vi "calculate_scanner_delays.vi"(8 "error in (no error)":errorcluster, 9 "position feedback data":T2, 10 "transformation parameters":T1={"scale factor"=1.0, "rotation angle"=0.0, "tilting angle"=0.0, "offset"=refnum}, 11 "TrajectoryDL091126GenericVoxel in":refnum<class "TrajectoryDL091126GenericVoxel.lvclass">) -> (0 "error out":errorcluster, 2 "calculated scanner delays":i32[](array[numeric]), 3 "TrajectoryDL091126GenericVoxel out":refnum<class "TrajectoryDL091126GenericVoxel.lvclass">)   [LabVIEW 2010, in "TrajectoryDL091126GenericVoxel.lvclass"]
uses:
  TrajectoryDL091126GenericVoxel.lvclass
  common/arrays/pixel_raw_data_array.ctl
  transformation_parameters.ctl
  common/classes/SpaceVector/SpaceVector/SpaceVector.lvclass
  <vilib>/Analysis/2dsp.llb/1D Cross Correlation (DBL).vi
  common/classes/ErrorController/ErrorController/class_data.vi
  <vilib>/Analysis/NI_AALPro.lvlib
  common/classes/ErrorController/ErrorController/ErrorController.lvclass
panel:
  out "Z scanner":dbl[](graph)
  out "Y scanner":dbl[](graph)
  out "X scanner":dbl[](graph)
  # "This VI uses cross-correlation to calculate the scanner delay.\n\nOverwrite this method in your Trajectory child class if you want to have your own algorithm."
  # "Cross-correlations between command and position-feedback signals"
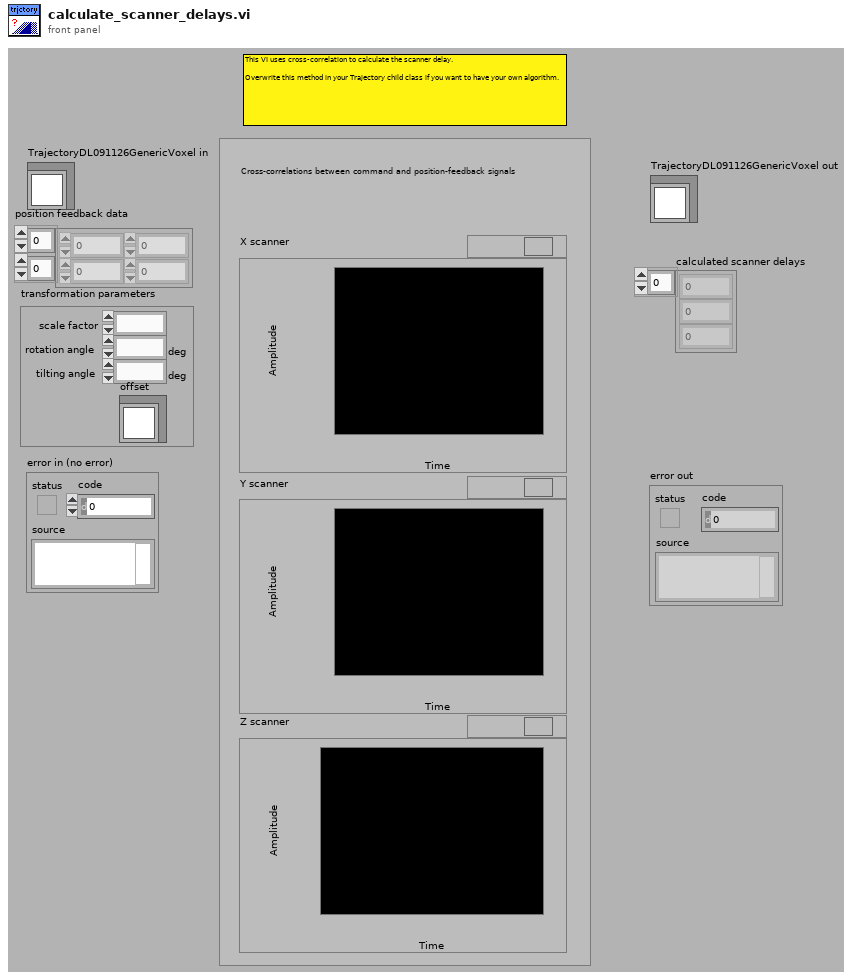
[diagram p1: front panel]
types:
  T1 = typedef "TrajectoryDL091126GenericVoxel.lvclass/transformation_parameters.ctl" = cluster{"scale factor":dbl, "rotation angle":dbl[unit], "tilting angle":dbl[unit], "offset":refnum<class "SpaceVector.lvclass">}
  T2 = typedef "pixel_raw_data_array.ctl" = dbl[][]
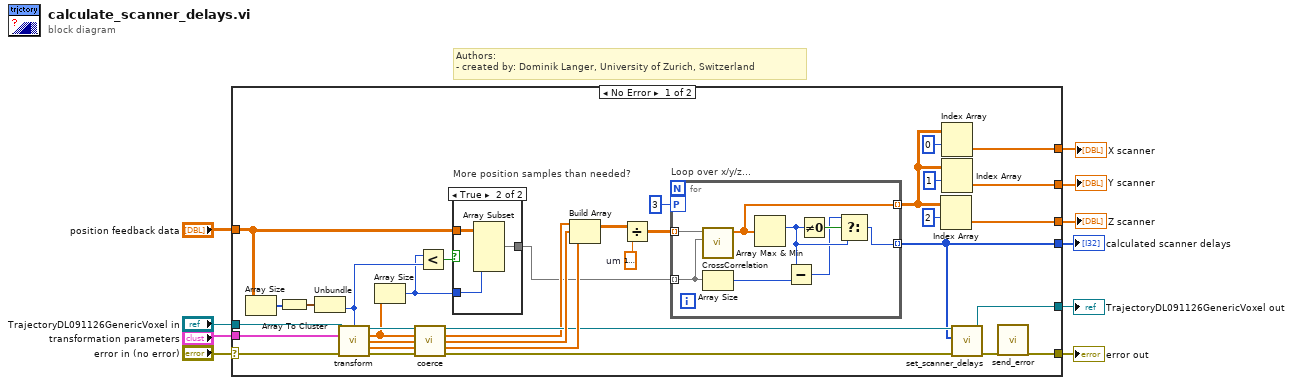
[diagram p0: block diagram]
diagram:
  # "Authors: \n- created by: Dominik Langer, University of Zurich, Switzerland"
  n1 = case shown="No Error" "error in (no error)" {
    selector: "error in (no error)" -> [w44 w59]
    tunnel: [w11 w59] -> w10
    tunnel: [w31 w58] -> w6
    tunnel: [w27 _] -> w3
    tunnel: [w30 _] -> w4
    tunnel: "position feedback data" -> [w18 _]
    tunnel: "TrajectoryDL091126GenericVoxel in" -> [w42 w58]
    tunnel: "transformation parameters" -> [w45 _]
    tunnel: [w26 _] -> w2
    tunnel: [w25 _] -> w1
    frame No Error {
      w34 = dbl[unit] 1e-06  # um
      n2 = Array Size(array=w18) -> (size(s)=w29:i32[])
      n3 = Array To Cluster(array=w29) -> (cluster=w28:cluster{"[0]":i32, "[1]":i32})
      n4 = Unbundle(w28) -> ("[1]"=w15:i32)  [unwired: 1 out]
      n5 = call-dynamic "transform.vi"("GenericTrajectory in"=w42, "number of pixels (all: -1)"=w15, "transformation parameters"=w45, "error in (no error)"=w44) -> ("GenericTrajectory out"=w43:refnum<class "TrajectoryDL091126GenericVoxel.lvclass">, "x coordinates"=w17:dbl[unit][], "y coordinates"=w40:dbl[unit][], "z coordinates"=w39:dbl[unit][], "error out"=w41:errorcluster)  [unwired: 7 in]
      n6 = Array Size(array=w17) -> (size(s)=w14:i32)
      n7 = call "coerce.vi"("GenericTrajectory in"=w43, "x coordinates in"=w17, "y coordinates in"=w40, "z coordinates in"=w39, "error in (no error)"=w41) -> ("GenericTrajectory out"=w32:refnum<class "TrajectoryDL091126GenericVoxel.lvclass">, "x coordinates out"=w20:dbl[unit][], "y coordinates out"=w38:dbl[unit][], "z coordinates out"=w37:dbl[unit][], "error out"=w33:errorcluster)  [unwired: 5 in, 1 out]
      n8 = Less?(x=w14, y=w15) -> (x < y?=w16:bool)
      n9 = case "More position samples than needed?" shown="True" w16 {
        tunnel: w18 -> [w46 w49]
        tunnel: [w46 w48] -> w13
        tunnel: w14 -> [_ w47]
        frame False {
        }
        frame True {
          n10 = Array Subset(array=w49, length (col)=w47) -> (w48:T2)  [unwired: 3 in]
        }
      }
      n11 = Build Array(w20, w38, w37) -> (w35:dbl[unit][][])
      n12 = Divide(x=w35, y=w34) -> (x/y=w36:dbl[][])
      n13 = for "Loop over x/y/z..." {
        tunnel: w36 -> [w54] mode=indexing
        tunnel: w13 -> [w57] mode=indexing
        tunnel: [w50] -> w30 mode=indexing
        workers-P: 3 -> [_]
        tunnel: [w55] -> w24 mode=indexing
        n14 = call-poly <vilib>:"CrossCorrelation.vi"("Y"=w57, "X"=w54) -> ("Rxy"=w55:dbl[])  [unwired: 8 in, 1 out]
        n15 = Array Size(array=w57) -> (size(s)=w56:i32)
        n16 = Array Max & Min(array=w55) -> (max index (indices)=w52:i32)  [unwired: 3 out]
        n17 = Subtract(x=w52, y=w56) -> (x-y=w51:i32)
        n18 = Not Equal To 0?(x=w52) -> (x != 0?=w53:bool)
        n19 = Select(t=w51, s=w53, f=w52) -> (s? t:f=w50:i32)
      }
      n20 = Index Array(array=w24, index (row)=2) -> (element=w25:dbl[])  [unwired: 1 in]
      n21 = Index Array(array=w24, index (row)=0) -> (element=w27:dbl[])  [unwired: 1 in]
      n22 = Index Array(array=w24, index (row)=1) -> (element=w26:dbl[])  [unwired: 1 in]
      n23 = call-dynamic "set_scanner_delays.vi"("error in (no error)"=w33, "scanner delays"=w30, "TrajectoryDL091126GenericVoxel in"=w32) -> ("error out"=w12:errorcluster, "TrajectoryDL091126GenericVoxel out"=w31:refnum<class "TrajectoryDL091126GenericVoxel.lvclass">)  [unwired: 7 in]
      n24 = call "send_error.vi"("error in (no error)"=w12) -> ("error out"=w11:errorcluster)  [unwired: 10 in]
    }
    frame Error {
    }
  }
  "error out" <- w10
  "TrajectoryDL091126GenericVoxel out" <- w6
  "calculated scanner delays" <- w4
  "X scanner" <- w3
  "Y scanner" <- w2
  "Z scanner" <- w1
